vi "Camera_Config_Global_Attributes.vi"(8 "error in (no error)":errorcluster, 10 "Refnum in":T2, 11 "input cluster":T1 {"SystemVersion" items=["Standard", "XL"]; "Overlay_Ring" items=["Session Data", "Extended Setup", "Buffer", "Camera", "Dispenser", "Stats", "Connections"]; "Flush Size" min=1; "Dispense Speed" min=1; "Rectangle 2"."Rotation" format="%.2f"; "Rectangle 2"."Left" scale=0.0..1024.0; "Rectangle 2"."Right" scale=0.0..1024.0; "Rectangle 1"."Rotation" format="%.2f"; "Rectangle 1"."Left" scale=0.0..1024.0; "Rectangle 1"."Right" scale=0.0..1024.0; "Max Framerate" min=1; "Overload threshold" min=1; "Image Save Queue Size" min=1; "Image Process Queue Size" min=1; "Empty start" min=1; "Sample size threshold" min=1; "Framerate" min=1; "Light intensity" scale=0.0..100.0}) -> (0 "error out":errorcluster, 2 "Refnum out":T2, 3 "input cluster out":T1 {"SystemVersion" items=["Standard", "XL"]; "Overlay_Ring" items=["Session Data", "Extended Setup", "Buffer", "Camera", "Dispenser", "Stats", "Connections"]; "Flush Size" min=1; "Dispense Speed" min=1; "Rectangle 2"."Rotation" format="%.2f"; "Rectangle 2"."Left" scale=0.0..1024.0; "Rectangle 2"."Right" scale=0.0..1024.0; "Rectangle 1"."Rotation" format="%.2f"; "Rectangle 1"."Left" scale=0.0..1024.0; "Rectangle 1"."Right" scale=0.0..1024.0; "Max Framerate" min=1; "Overload threshold" min=1; "Image Save Queue Size" min=1; "Image Process Queue Size" min=1; "Empty start" min=1; "Sample size threshold" min=1; "Framerate" min=1; "Light intensity" scale=0.0..100.0})   [LabVIEW 2022 SP3]
uses:
  controls/Data.ctl
  <vilib>/userdefined/High Color/IMAQdx.ctl
  <vilib>/vision/Image Controls.llb/IMAQ Image.ctl
  <resource>/objmgr/imaqdx.rc
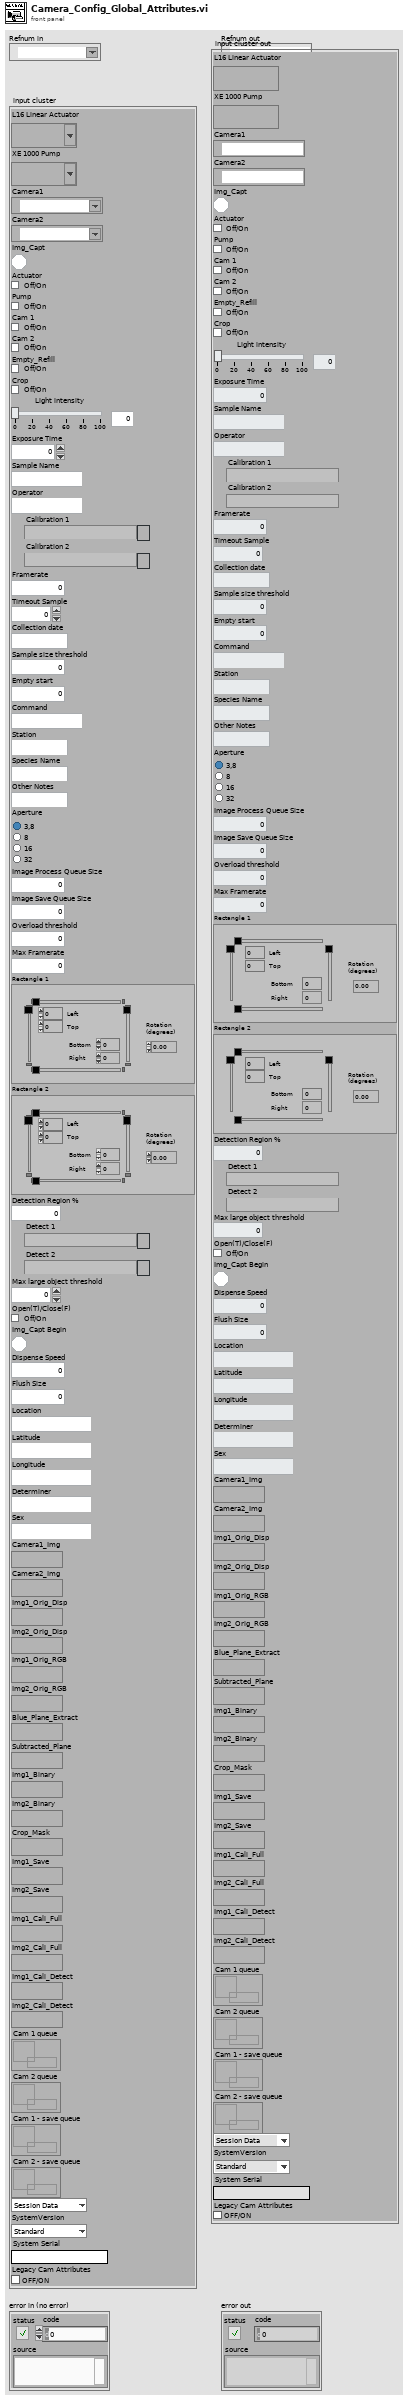
[diagram p1: front panel]
types:
  T1 = typedef "Data.ctl" = cluster{"L16 Linear Actuator":refnum<visa-resource-name>, "XE 1000 Pump":refnum<visa-resource-name>, "Camera1":T2, "Camera2":T2, "Img_Capt":bool, "Actuator":bool, "Pump":bool, "Cam 1":bool, "Cam 2":bool, "Empty_Refill":bool, "Crop":bool, "Light intensity":i32, "Exposure Time":dbl, "Sample Name":string, "Operator":string, "Calibration 1":path, "Calibration 2":path, "Framerate":i32, "Timeout Sample":i32, "Collection date":string, "Sample size threshold":i32, "Empty start":u32, "Command":string, "Station":string, "Species Name":string, "Other Notes":string, "Aperture":enum32{"Item 0", "Item 1", "Item 2", "Item 3"}, "Image Process Queue Size":i32, "Image Save Queue Size":i32, "Overload threshold":i32, "Max Framerate":i32, "Rectangle 1":T3, "Rectangle 2":T3, "Detection Region %":dbl, "Detect 1":path, "Detect 2":path, "Max large object threshold":i32, "Open(T)/Close(F)":bool, "Img_Capt Begin":bool, "Dispense Speed":i32, "Flush Size":i32, "Location":string, "Latitude":string, "Longitude":string, "Determiner":string, "Sex":string, "Camera1_Img":T4, "Camera2_Img":T4, "Img1_Orig_Disp":T4, "Img2_Orig_Disp":T4, "Img1_Orig_RGB":T4, "Img2_Orig_RGB":T4, "Blue_Plane_Extract":T4, "Subtracted_Plane":T4, "Img1_Binary":T4, "Img2_Binary":T4, "Crop_Mask":T4, "Img1_Save":T4, "Img2_Save":T4, "Img1_Cali_Full":T4, "Img2_Cali_Full":T4, "Img1_Cali_Detect":T4, "Img2_Cali_Detect":T4, "Cam 1 queue":refnum<queue>, "Cam 2 queue":refnum<queue>, "Cam 1 - save queue":refnum<queue>, "Cam 2 - save queue":refnum<queue>, "Overlay_Ring":u16, "SystemVersion":u16, "System Serial":string, "Legacy Cam Attributes":bool}
  T2 = typedef "IMAQdx.ctl" = refnum<k21>
  T3 = typedef "IMAQ Rectangle" = cluster{"Left":i32, "Top":i32, "Right":i32, "Bottom":i32, "Rotation":dbl}
  T4 = typedef "IMAQ Image.ctl" = refnum<image>
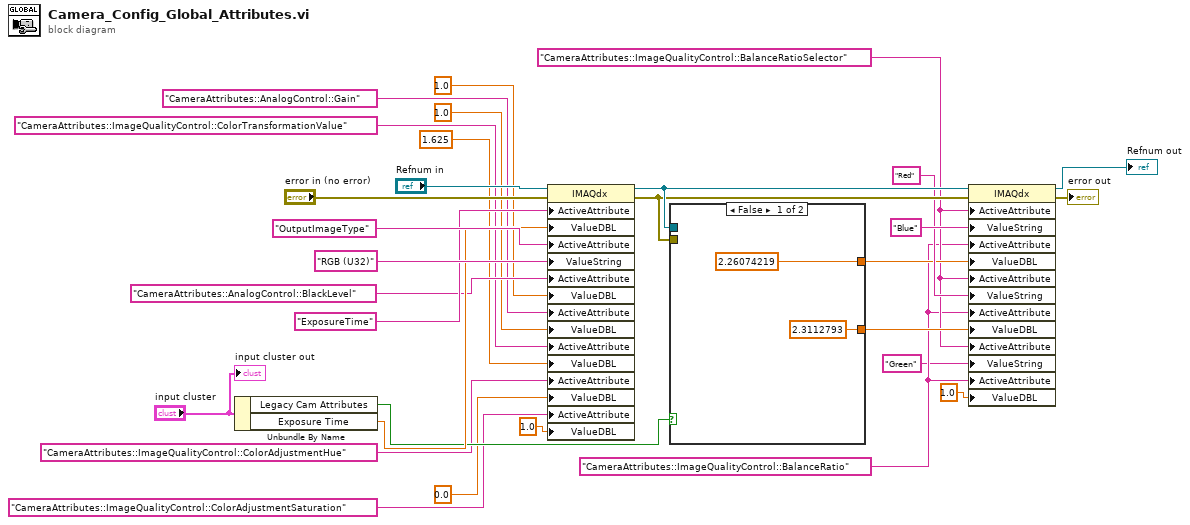
[diagram p0: block diagram]
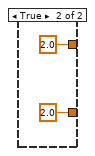
[diagram p2: hidden frame]
diagram:
  w3 = "CameraAttributes::ImageQualityControl::BalanceRatio" ("ActiveAttribute")
  w4 = "CameraAttributes::ImageQualityControl::BalanceRatioSelector" ("ActiveAttribute")
  n1 = Unbundle By Name("input cluster") -> ("Legacy Cam Attributes"=w21:bool, "Exposure Time"=w25:dbl)
  n2 = property class="IMAQdx"(reference="Refnum in", error in="error in (no error)", "ActiveAttribute"="ExposureTime", "ValueDBL"=w25, "ActiveAttribute"="OutputImageType", "ValueString"="RGB (U32)", "ActiveAttribute"="CameraAttributes::AnalogControl::BlackLevel", "ValueDBL"=1.0, "ActiveAttribute"="CameraAttributes::AnalogControl::Gain", "ValueDBL"=1.0, "ActiveAttribute"="CameraAttributes::ImageQualityControl::ColorTransformationValue", "ValueDBL"=1.625, "ActiveAttribute"="CameraAttributes::ImageQualityControl::ColorAdjustmentHue", "ValueDBL"=0.0, "ActiveAttribute"="CameraAttributes::ImageQualityControl::ColorAdjustmentSaturation", "ValueDBL"=1.0) -> (reference out=w23:T2, error out=w22:errorcluster)
  n3 = case shown="False" w21 {
    tunnel: w23 -> [_ _]
    tunnel: w22 -> [_ _]
    tunnel: [2.26074219 ("ValueDBL") 2.0 ("ValueDBL")] -> w16
    tunnel: [2.3112793 ("ValueDBL") 2.0 ("ValueDBL")] -> w15
    frame False {
    }
    frame True {
    }
  }
  n4 = property class="IMAQdx"(reference=w23, error in=w22, "ActiveAttribute"=w4, "ValueString"="Blue", "ActiveAttribute"=w3, "ValueDBL"=w16, "ActiveAttribute"=w4, "ValueString"="Red", "ActiveAttribute"=w3, "ValueDBL"=w15, "ActiveAttribute"=w4, "ValueString"="Green", "ActiveAttribute"=w3, "ValueDBL"=1.0) -> (reference out=→"Refnum out":T2, error out=→"error out":errorcluster)
  "input cluster out" <- "input cluster"
